vi "Write_CmdSingleParam.vi"(8 "error in (no error)":errorcluster, 9 "Param":i32, 10 "Command":enum16{"SA", "GT", "SI", "SL", "ST", "CT"}(ring), 11 "Multiplexer_Opmux in":refnum<class "Multiplexer_Opmux.lvclass">) -> (0 "error out":errorcluster, 3 "Multiplexer_Opmux out":refnum<class "Multiplexer_Opmux.lvclass">)   [LabVIEW 2014, in "Multiplexer_Opmux.lvclass"]
uses:
  Multiplexer_Opmux.lvclass
  Multiplexer_Opmux.lvclass/Multiplexer_Opmux.ctl
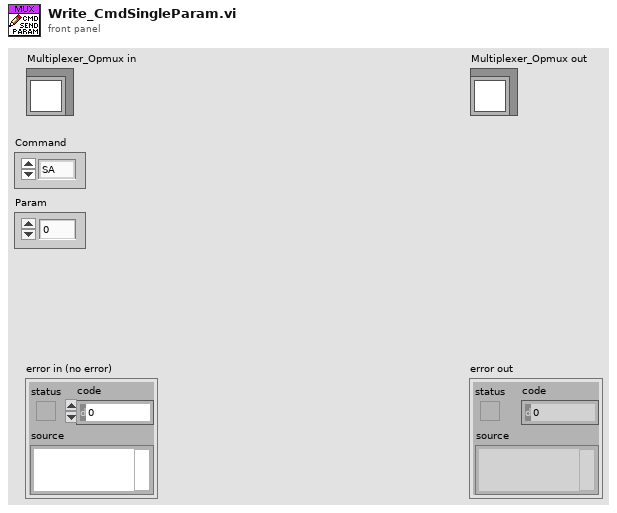
[diagram p1: front panel]
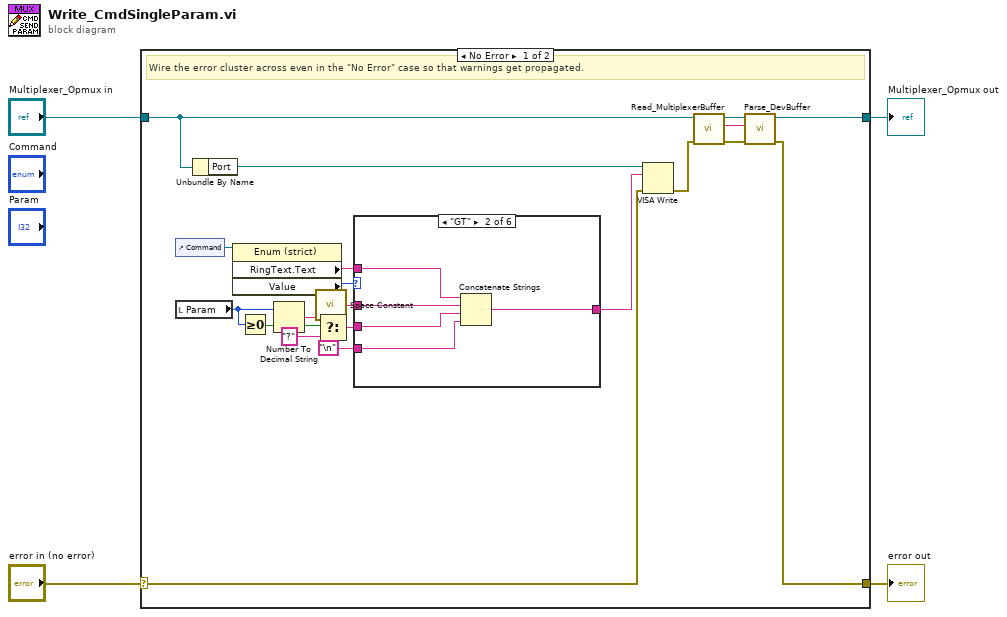
[diagram p0: block diagram]
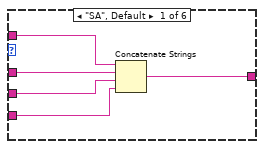
[diagram p2: hidden frame]
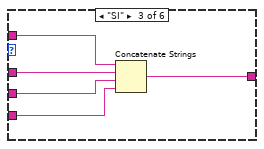
[diagram p3: hidden frame]
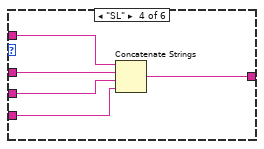
[diagram p4: hidden frame]
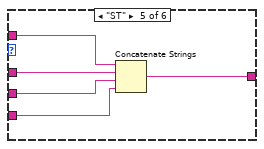
[diagram p5: hidden frame]
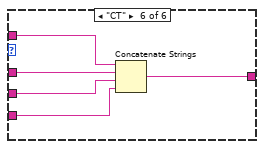
[diagram p6: hidden frame]
diagram:
  n1 = case shown="No Error" "error in (no error)" {
    selector: "error in (no error)" -> [w10 w56]
    tunnel: [w5 w56] -> w3
    tunnel: [w8 w55] -> w1
    tunnel: "Multiplexer_Opmux in" -> [w11 w55]
    frame No Error {
      # "Wire the error cluster across even in the \"No Error\" case so that warnings get propagated."
      n2 = control-ref of="Command"() -> (w14:refnum<vi>)
      n3 = local read "Param"() -> (w24:i32)
      n4 = Unbundle By Name(w11) -> ("Port"=w13:refnum<visa-resource-name>)
      n5 = property class="Enum (strict)"(reference=w14) -> ("RingText.Text"=w16:string, "Value"=w15:enum16{"SA", "GT", "SI", "SL", "ST", "CT"})  [unwired: 1 in, 2 out]
      n6 = Greater Or Equal To 0?(x=w24) -> (x >= 0?=w23:bool)
      n7 = Number To Decimal String(number=w24) -> (decimal integer string=w21:string)  [unwired: 1 in]
      n8 = call <vilib>:"Space Constant.vi"() -> ("String"=w18:string)
      n9 = Select(t=w21, s=w23, f="?") -> (s? t:f=w20:string)
      n10 = case shown="\"GT\"" w15 {
        tunnel: w16 -> [w28 w33 w38 w43 w48 w53]
        tunnel: [w25 w30 w35 w40 w45 w50] -> w17
        tunnel: w18 -> [w29 w34 w39 w44 w49 w54]
        tunnel: "\n" -> [w26 w31 w36 w41 w46 w51]
        tunnel: w20 -> [w27 w32 w37 w42 w47 w52]
        frame "SA", Default {
          n11 = Concatenate Strings(w28, w29, w27, w26) -> (w25:string)
        }
        frame "GT" {
          n12 = Concatenate Strings(w33, w34, w32, w31) -> (w30:string)
        }
        frame "SI" {
          n13 = Concatenate Strings(w38, w39, w37, w36) -> (w35:string)
        }
        frame "SL" {
          n14 = Concatenate Strings(w43, w44, w42, w41) -> (w40:string)
        }
        frame "ST" {
          n15 = Concatenate Strings(w48, w49, w47, w46) -> (w45:string)
        }
        frame "CT" {
          n16 = Concatenate Strings(w53, w54, w52, w51) -> (w50:string)
        }
      }
      n17 = VISA Write(VISA resource name=w13, write buffer=w17, error in (no error)=w10) -> (error out=w9:errorcluster)  [unwired: 2 out]
      n18 = call-dynamic "Read_MultiplexerBuffer.vi"("error in (no error)"=w9, "Multiplexer_Opmux in"=w11) -> ("error out"=w7:errorcluster, "BufferOut"=w6:string, "Multiplexer_Opmux out"=w12:refnum<class "Multiplexer_Opmux.lvclass">)  [unwired: 7 in]
      n19 = call-dynamic "Parse_DevBuffer.vi"("error in (no error)"=w7, "searchFor"=w6, "Multiplexer_Opmux in"=w12) -> ("error out"=w5:errorcluster, "Multiplexer_Opmux out"=w8:refnum<class "Multiplexer_Opmux.lvclass">)  [unwired: 6 in, 1 out]
    }
    frame Error {
    }
  }
  "error out" <- w3
  "Multiplexer_Opmux out" <- w1
